vi "GearG&D.vi"(2 "Grab":bool) -> ()   [LabVIEW 2016]
uses:
  <vilib>/Rock Robotics/WPI/Solenoid/WPI_SolenoidValue.ctl
  <vilib>/Rock Robotics/WPI/Solenoid/WPI_SolenoidSetEnum.vi
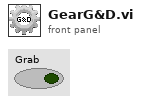
[diagram p1: front panel]
types:
  T1 = typedef "WPI_SolenoidValue.ctl" = enum16{"Off", "On", "Forward", "Reverse"}
  T2 = typedef "WPI_SolenoidDevRef.ctl" = cluster{"DevStatus":errorcluster, "Pneumatics Control Module":u8, "Forward Solenoid Channel":T3, "Reverse Solenoid Channel":T3}
  T3 = typedef "WPI_SolenoidChannel.ctl" = enum8{"Solenoid 0", "Solenoid 1", "Solenoid 2", "Solenoid 3", "Solenoid 4", "Solenoid 5", "Solenoid 6", "Solenoid 7", "Invalid"}
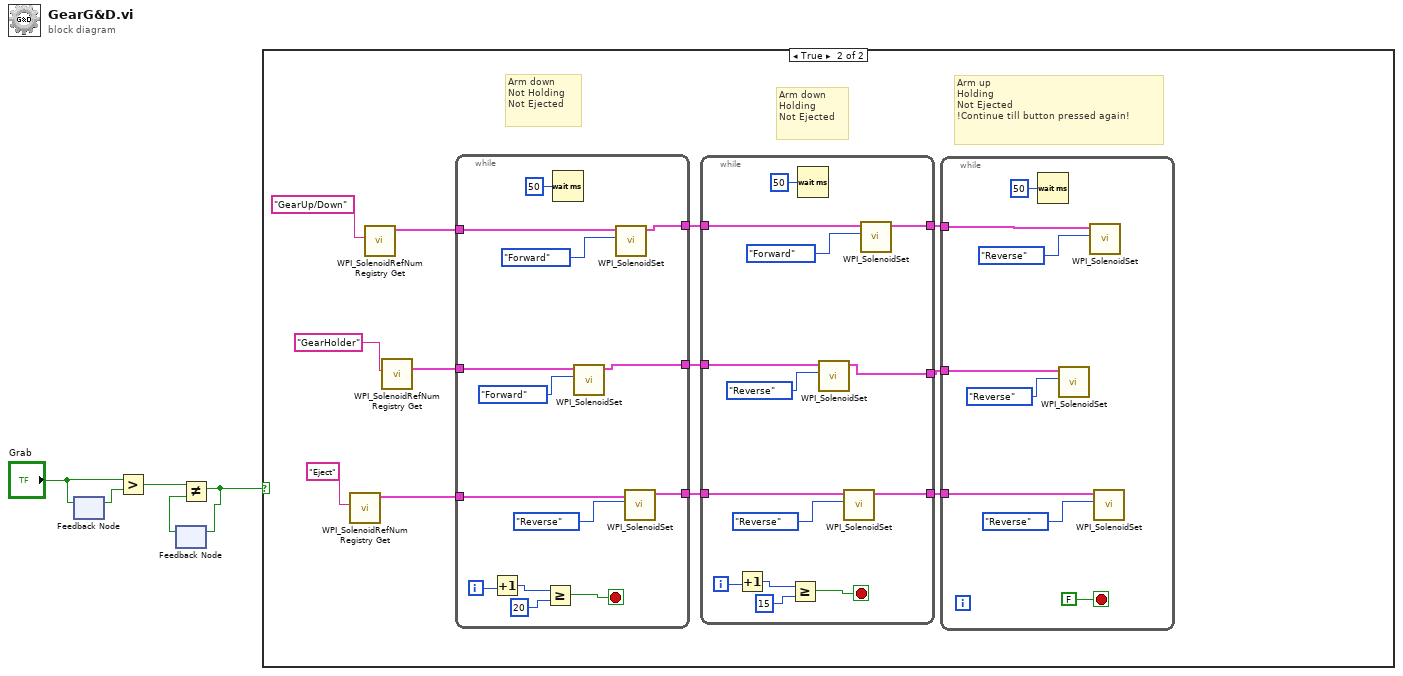
[diagram p0: block diagram]
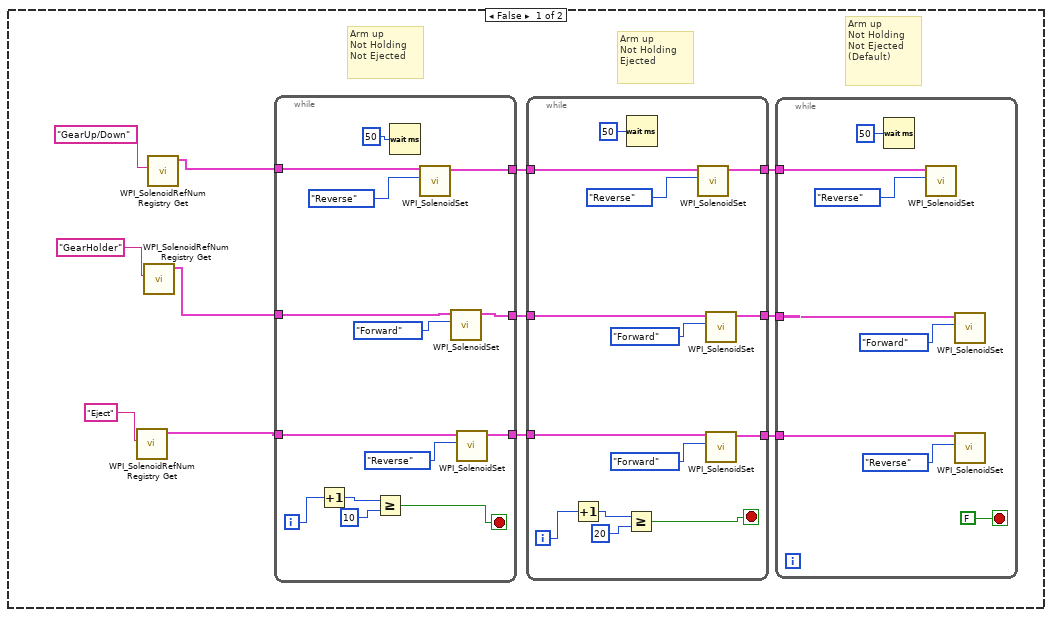
[diagram p2: hidden frame]
diagram:
  n1 = feedback #1() -> (w4:bool)  [unwired: 1 in]
  n2 = feedback-in #1("Grab") -> ()
  n3 = Greater?(x="Grab", y=w4) -> (0:w5:bool)
  n4 = feedback #2() -> (w3:bool)  [unwired: 1 in]
  n5 = Not Equal?(x=w5, y=w3) -> (x != y?=w1:bool)
  n6 = feedback-in #2(w1) -> ()
  n7 = case shown="True" w1 {
    frame False {
      # "Arm up\nNot Holding\nNot Ejected\n(Default)"
      # "Arm up\nNot Holding\nEjected"
      # "Arm up\nNot Holding\nNot Ejected"
      n8 = call <vilib>:"WPI_SolenoidRefNum Registry Get.vi"("refnum name"="Eject") -> ("SolenoidDevRef"=w6:T2)  [unwired: 9 in, 1 out]
      n9 = call <vilib>:"WPI_SolenoidRefNum Registry Get.vi"("refnum name"="GearHolder") -> ("SolenoidDevRef"=w7:T2)  [unwired: 9 in, 1 out]
      n10 = call <vilib>:"WPI_SolenoidRefNum Registry Get.vi"("refnum name"="GearUp/Down") -> ("SolenoidDevRef"=w8:T2)  [unwired: 9 in, 1 out]
      n11 = while {
        tunnel: [w47] -> w14
        tunnel: [w46] -> w13
        tunnel: w7 -> [w44]
        tunnel: w6 -> [w43]
        tunnel: w8 -> [w41]
        tunnel: [w40] -> w10
        i -> [w49]
        stop <- w48 stop-if-true
        n12 = Increment(x=w49) -> (x+1=w51:i32)
        n13 = Greater Or Equal?(x=w51, y=10) -> (x >= y?=w48:bool)
        n14 = Wait (ms)(milliseconds to wait=u32 50) -> ()  [unwired: 1 out]
        n15 = call-poly <vilib>:"WPI_SolenoidSet.vi"("Value"=WPI_SolenoidValue."Reverse", "SolenoidDevRef"=w41) -> ("SolenoidDevRef"=w40:T2)  [unwired: 8 in, 1 out]
        n16 = call-poly <vilib>:"WPI_SolenoidSet.vi"("Value"=WPI_SolenoidValue."Forward", "SolenoidDevRef"=w44) -> ("SolenoidDevRef"=w46:T2)  [unwired: 8 in, 1 out]
        n17 = call-poly <vilib>:"WPI_SolenoidSet.vi"("Value"=WPI_SolenoidValue."Reverse", "SolenoidDevRef"=w43) -> ("SolenoidDevRef"=w47:T2)  [unwired: 8 in, 1 out]
      }
      n18 = while {
        tunnel: w14 -> [w37]
        tunnel: w13 -> [w36]
        tunnel: [w31] -> w12
        tunnel: [w30] -> w11
        tunnel: w10 -> [w27]
        tunnel: [w26] -> w9
        i -> [w33]
        stop <- w32 stop-if-true
        n19 = Increment(x=w33) -> (x+1=w35:i32)
        n20 = Greater Or Equal?(x=w35, y=20) -> (x >= y?=w32:bool)
        n21 = Wait (ms)(milliseconds to wait=u32 50) -> ()  [unwired: 1 out]
        n22 = call-poly <vilib>:"WPI_SolenoidSet.vi"("Value"=WPI_SolenoidValue."Reverse", "SolenoidDevRef"=w27) -> ("SolenoidDevRef"=w26:T2)  [unwired: 8 in, 1 out]
        n23 = call-poly <vilib>:"WPI_SolenoidSet.vi"("Value"=WPI_SolenoidValue."Forward", "SolenoidDevRef"=w36) -> ("SolenoidDevRef"=w30:T2)  [unwired: 8 in, 1 out]
        n24 = call-poly <vilib>:"WPI_SolenoidSet.vi"("Value"=WPI_SolenoidValue."Forward", "SolenoidDevRef"=w37) -> ("SolenoidDevRef"=w31:T2)  [unwired: 8 in, 1 out]
      }
      n25 = while {
        tunnel: w12 -> [w23]
        tunnel: w11 -> [w22]
        tunnel: w9 -> [w18]
        stop <- FALSE stop-if-true
        n26 = Wait (ms)(milliseconds to wait=u32 50) -> ()  [unwired: 1 out]
        n27 = call-poly <vilib>:"WPI_SolenoidSet.vi"("Value"=WPI_SolenoidValue."Reverse", "SolenoidDevRef"=w18) -> ()  [unwired: 8 in, 2 out]
        n28 = call-poly <vilib>:"WPI_SolenoidSet.vi"("Value"=WPI_SolenoidValue."Forward", "SolenoidDevRef"=w22) -> ()  [unwired: 8 in, 2 out]
        n29 = call-poly <vilib>:"WPI_SolenoidSet.vi"("Value"=WPI_SolenoidValue."Reverse", "SolenoidDevRef"=w23) -> ()  [unwired: 8 in, 2 out]
      }
    }
    frame True {
      # "Arm up\nHolding\nNot Ejected\n!Continue till button pressed again!"
      # "Arm down\nHolding\nNot Ejected"
      # "Arm down\nNot Holding\nNot Ejected"
      n30 = call <vilib>:"WPI_SolenoidRefNum Registry Get.vi"("refnum name"="Eject") -> ("SolenoidDevRef"=w56:T2)  [unwired: 9 in, 1 out]
      n31 = call <vilib>:"WPI_SolenoidRefNum Registry Get.vi"("refnum name"="GearUp/Down") -> ("SolenoidDevRef"=w64:T2)  [unwired: 9 in, 1 out]
      n32 = call <vilib>:"WPI_SolenoidRefNum Registry Get.vi"("refnum name"="GearHolder") -> ("SolenoidDevRef"=w62:T2)  [unwired: 9 in, 1 out]
      n33 = while {
        tunnel: w64 -> [w101]
        tunnel: w62 -> [w100]
        tunnel: [w92] -> w61
        tunnel: [w91] -> w60
        tunnel: w56 -> [w89]
        tunnel: [w88] -> w55
        i -> [w97]
        stop <- w94 stop-if-true
        n34 = Increment(x=w97) -> (x+1=w95:i32)
        n35 = Greater Or Equal?(x=w95, y=20) -> (x >= y?=w94:bool)
        n36 = Wait (ms)(milliseconds to wait=u32 50) -> ()  [unwired: 1 out]
        n37 = call-poly <vilib>:"WPI_SolenoidSet.vi"("Value"=WPI_SolenoidValue."Forward", "SolenoidDevRef"=w100) -> ("SolenoidDevRef"=w91:T2)  [unwired: 8 in, 1 out]
        n38 = call-poly <vilib>:"WPI_SolenoidSet.vi"("Value"=WPI_SolenoidValue."Forward", "SolenoidDevRef"=w101) -> ("SolenoidDevRef"=w92:T2)  [unwired: 8 in, 1 out]
        n39 = call-poly <vilib>:"WPI_SolenoidSet.vi"("Value"=WPI_SolenoidValue."Reverse", "SolenoidDevRef"=w89) -> ("SolenoidDevRef"=w88:T2)  [unwired: 8 in, 1 out]
      }
      n40 = while {
        tunnel: w61 -> [w87]
        tunnel: w60 -> [w86]
        tunnel: [w78] -> w59
        tunnel: [w77] -> w58
        tunnel: w55 -> [w75]
        tunnel: [w74] -> w54
        i -> [w83]
        stop <- w80 stop-if-true
        n41 = Increment(x=w83) -> (x+1=w81:i32)
        n42 = Greater Or Equal?(x=w81, y=15) -> (x >= y?=w80:bool)
        n43 = Wait (ms)(milliseconds to wait=u32 50) -> ()  [unwired: 1 out]
        n44 = call-poly <vilib>:"WPI_SolenoidSet.vi"("Value"=WPI_SolenoidValue."Reverse", "SolenoidDevRef"=w86) -> ("SolenoidDevRef"=w77:T2)  [unwired: 8 in, 1 out]
        n45 = call-poly <vilib>:"WPI_SolenoidSet.vi"("Value"=WPI_SolenoidValue."Reverse", "SolenoidDevRef"=w75) -> ("SolenoidDevRef"=w74:T2)  [unwired: 8 in, 1 out]
        n46 = call-poly <vilib>:"WPI_SolenoidSet.vi"("Value"=WPI_SolenoidValue."Forward", "SolenoidDevRef"=w87) -> ("SolenoidDevRef"=w78:T2)  [unwired: 8 in, 1 out]
      }
      n47 = while {
        tunnel: w59 -> [w73]
        tunnel: w58 -> [w72]
        tunnel: w54 -> [w67]
        stop <- FALSE stop-if-true
        n48 = Wait (ms)(milliseconds to wait=u32 50) -> ()  [unwired: 1 out]
        n49 = call-poly <vilib>:"WPI_SolenoidSet.vi"("Value"=WPI_SolenoidValue."Reverse", "SolenoidDevRef"=w72) -> ()  [unwired: 8 in, 2 out]
        n50 = call-poly <vilib>:"WPI_SolenoidSet.vi"("Value"=WPI_SolenoidValue."Reverse", "SolenoidDevRef"=w73) -> ()  [unwired: 8 in, 2 out]
        n51 = call-poly <vilib>:"WPI_SolenoidSet.vi"("Value"=WPI_SolenoidValue."Reverse", "SolenoidDevRef"=w67) -> ()  [unwired: 8 in, 2 out]
      }
    }
  }
